vi "CTRE_PigeonIMU_UpdateUsage.vi"(10 "Usage":T3 items=["Defaul"=0, "ConnectCAN"=1, "ConnectTalonSRX"=2, "GetCompass"=134217728, "GetYPR"=268435456, "GetFused"=536870912, "GetAccel"=1073741824, "TempComp"=2147483648], 11 "PigeonIMUDevRef":T1={"DeviceStatus"={"status"=FALSE, "code"=0, "source"=""}, "Device Number"=0, "Type"=352321536, "Device ID"=0, "Handle"=0, "UsageFrame"=0, "Library Path"=path ""} {"Type" items=["CAN"=352321536, "TalonSRX"=33554432]}) -> (3 "PigeonIMUDevRef":T1={"DeviceStatus"={"status"=FALSE, "code"=0, "source"=""}, "Device Number"=0, "Type"=352321536, "Device ID"=0, "Handle"=0, "UsageFrame"=0, "Library Path"=path ""} {"Type" items=["CAN"=352321536, "TalonSRX"=33554432]})   [LabVIEW 2020]
uses:
  <vilib>/Rock Robotics/WPI/ThirdParty/Phoenix-LabVIEW/Pigeon IMU/CTRE_PigeonIMU_DeviceRef.ctl
  <vilib>/Rock Robotics/WPI/ThirdParty/Phoenix-LabVIEW/Pigeon IMU/CTRE_PigeonIMU_ConnectionType.ctl
  <vilib>/Rock Robotics/WPI/ThirdParty/Phoenix-LabVIEW/Pigeon IMU/CTRE_PigeonIMU_UsageTypes.ctl
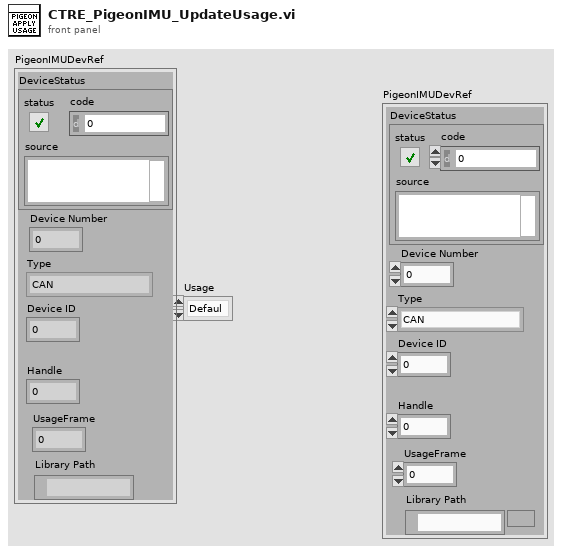
[diagram p1: front panel]
types:
  T1 = typedef "CTRE_PigeonIMU_DeviceRef.ctl" = cluster{"DeviceStatus":errorcluster, "Device Number":u8, "Type":T2, "Device ID":u32, "Handle":u64, "UsageFrame":u32, "Library Path":path}
  T2 = typedef "CTRE_PigeonIMU_ConnectionType.ctl" = u32
  T3 = typedef "CTRE_PigeonIMU_UsageTypes.ctl" = u32
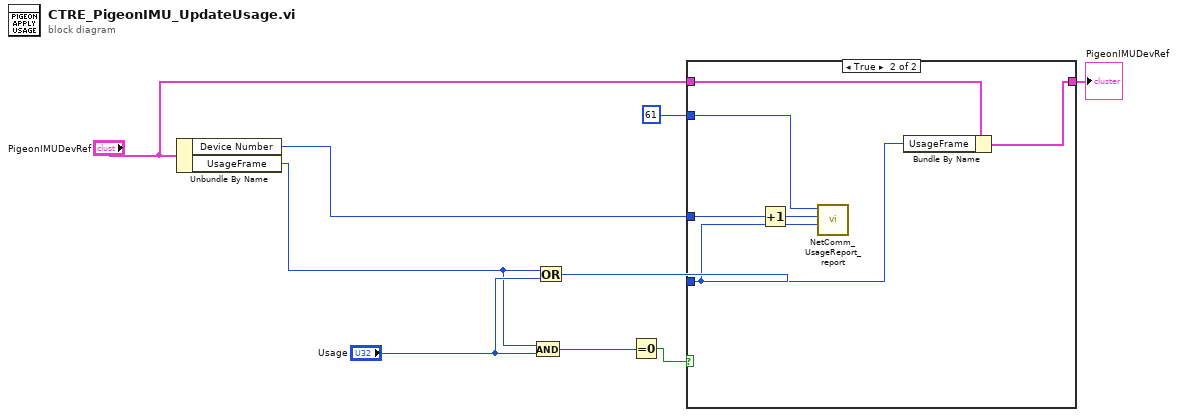
[diagram p0: block diagram]
diagram:
  n1 = Unbundle By Name("PigeonIMUDevRef") -> ("Device Number"=w5:u8, "UsageFrame"=w1:u32)
  n2 = And(x=w1, y="Usage") -> (x .and. y?=w8:T3)
  n3 = Or(x=w1, y="Usage") -> (x .or. y?=w7:T3)
  n4 = Equal To 0?(x=w8) -> (x = 0?=w9:bool)
  n5 = case shown="True" w9 {
    tunnel: 61 -> [_ w16]
    tunnel: w5 -> [_ w14]
    tunnel: w7 -> [_ w11]
    tunnel: "PigeonIMUDevRef" -> [w10 w13]
    tunnel: [w10 w12] -> w2
    frame False {
    }
    frame True {
      n6 = Increment(x=w14) -> (x+1=w15:u8)
      n7 = call <vilib>:"NetComm_UsageReport_report.vi"("Context"=w11, "Instance Number"=w15, "Resource Type"=w16) -> ()  [unwired: 9 in]
      n8 = Bundle By Name(cluster=w13, "UsageFrame"=w11) -> (w12:T1)
    }
  }
  "PigeonIMUDevRef" <- w2
